vi "DT_Triangle Manager_Remove Ghost.vi"(10 "update adj tri?":bool, 11 "Triangles In":i32[][](array[numeric])) -> (3 "Triangles Out":i32[][](array[numeric]))   [LabVIEW 2020, in "NI_AAL_Geometry.lvlib"]
uses:
  <vilib>/Analysis/NI_AAL_Geometry.lvlib
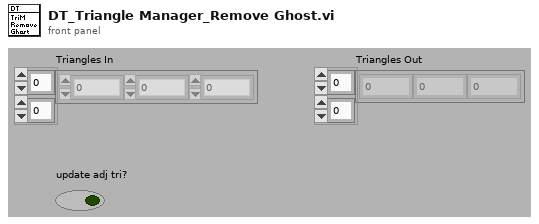
[diagram p1: front panel]
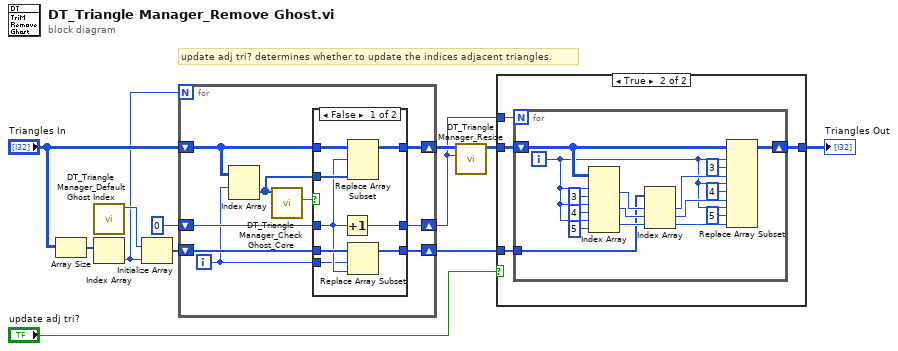
[diagram p0: block diagram]
diagram:
  # "update adj tri? determines whether to update the indices adjacent triangles."
  n1 = Array Size(array="Triangles In") -> (size(s)=w9:i32[])
  n2 = call <vilib>:"DT_Triangle Manager_Default Ghost Index.vi"() -> ("ghost index"=w8:i32)  [unwired: 11 out]
  n3 = Index Array(array=w9) -> (element=w3:i32)  [unwired: 1 in]
  n4 = Initialize Array(w8, w3) -> (w7:i32[])
  n5 = for {
    N: w3 -> [_]
    shift-right: [w21] -> w11
    shift-left: "Triangles In" -> [w16]
    shift-right: [w19] -> w2
    shift-left: 0 -> [w20]
    shift-right: [w17] -> w5
    shift-left: w7 -> [w18]
    i -> [w15]
    n6 = Index Array(array=w16, index (row)=w15) -> (element=w14:i32[])  [unwired: 1 in]
    n7 = call <vilib>:"DT_Triangle Manager_Check Ghost_Core.vi"("Triangle"=w14) -> ("ghost tri?"=w13:bool)  [unwired: 10 out]
    n8 = case shown="False" w13 {
      tunnel: w16 -> [w29 w32]
      tunnel: [w28 w32] -> w21
      tunnel: w20 -> [w24 w31]
      tunnel: w14 -> [w27 _]
      tunnel: [w26 w31] -> w19
      tunnel: w18 -> [w25 w30]
      tunnel: [w23 w30] -> w17
      tunnel: w15 -> [w22 _]
      frame False {
        n9 = Increment(x=w24) -> (x+1=w26:i32)
        n10 = Replace Array Subset(array=w29, new element=w27, index (row)=w24) -> (w28:i32[][])  [unwired: 1 in]
        n11 = Replace Array Subset(array=w25, new element=w24, index=w22) -> (w23:i32[])
      }
      frame True {
      }
    }
  }
  n12 = call <vilib>:"DT_Triangle Manager_Resize.vi"("# of triangles"=w2, "Triangles In"=w11) -> ("Triangles Out"=w1:i32[][])  [unwired: 9 out]
  n13 = case shown="True" "update adj tri?" {
    tunnel: w1 -> [w33 w36]
    tunnel: w5 -> [_ w37]
    tunnel: [w33 w35] -> w4
    tunnel: w2 -> [_ w34]
    frame False {
    }
    frame True {
      n14 = for {
        N: w34 -> [_]
        tunnel: w37 -> [w42]
        shift-right: [w44] -> w35
        shift-left: w36 -> [w43]
        i -> [w41]
        n15 = Index Array(array=w43, index (row) #1=w41, index (col) #1=3 ("disabled index (col)"), index (row) #2=w41, index (col) #2=4 ("disabled index (col)"), index (row) #3=w41, index (col) #3=5 ("disabled index (col)")) -> (element #1=w53:i32, element #2=w52:i32, element #3=w51:i32)
        n16 = Index Array(array=w42, index #1=w53, index #2=w52, index #3=w51) -> (element #1=w49:i32, element #2=w47:i32, element #3=w46:i32)
        n17 = Replace Array Subset(array=w43, new element #1=w49, index (row) #1=w41, index (col) #1=3 ("disabled index (col)"), new element #2=w47, index (row) #2=w41, index (col) #2=4 ("disabled index (col)"), new element #3=w46, index (row) #3=w41, index (col) #3=5 ("disabled index (col)")) -> (w44:i32[][])
      }
    }
  }
  "Triangles Out" <- w4
